vi "APC_init.vi"() -> (0 "error out":errorcluster)   [LabVIEW 2018]
uses:
  <vilib>/Utility/error.llb/Error Cluster From Error Code.vi
  <vilib>/ErrorRing/Error Ring.xnode
panel:
  # "The semaphore handshake with the APC control program is setup\nin a very simple way. A file \"C:\\Users\\Public\\SystemWillShutdown\"\nis created when there is a problem with the power network. This file\nis not deleted by APC control program and must be deleted from\nthis program."
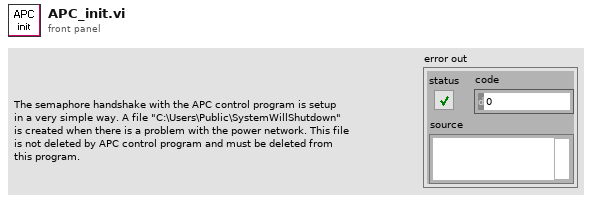
[diagram p1: front panel]
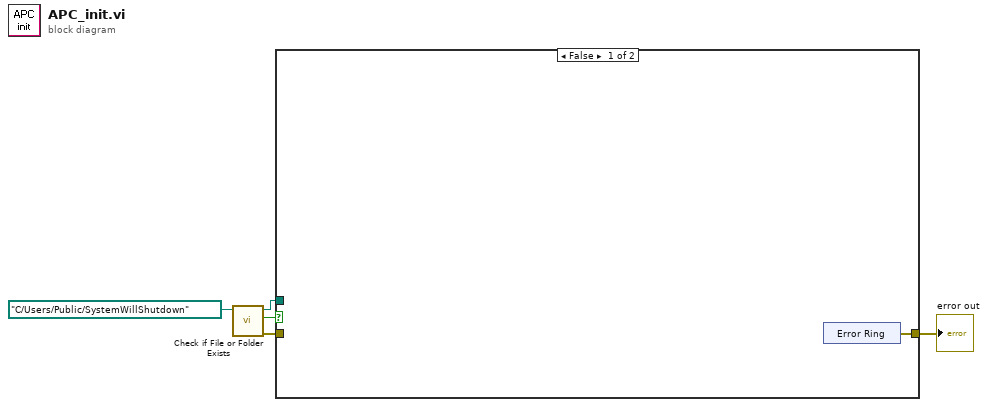
[diagram p0: block diagram]
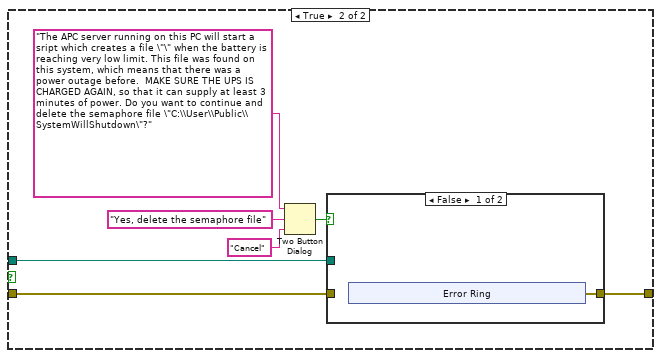
[diagram p2: hidden frame]
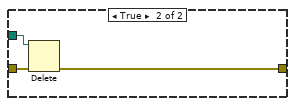
[diagram p3: hidden frame]
diagram:
  n1 = call <vilib>:"Check if File or Folder Exists.vi"("path"=path "C:/Users/Public/SystemWillShutdown" ("path (use dialog)")) -> ("error out"=w3:errorcluster, "file or folder exists?"=w4:bool, "dup path"=w2:path)  [unwired: 8 in]
  n2 = case shown="False" w4 {
    tunnel: w3 -> [_ w9]
    tunnel: w2 -> [_ w10]
    tunnel: [w6 w8] -> w1
    frame False {
      n3 = xnode "Error Ring"() -> ("error out"=w6:errorcluster)
    }
    frame True {
      n4 = Two Button Dialog(message="The APC server running on this PC will start a sript which creates a file \"\" when the battery is reaching very low limit. This file was found on this system, which means that there was a power outage before.  MAKE SURE THE UPS IS CHARGED AGAIN, so that it can supply at least 3 minutes of power. Do you want to continue and delete the semaphore file \"C:\\User\\Public\\SystemWillShutdown\"?", 1:"Cancel" ("F button name (\"Cancel\")"), 2:"Yes, delete the semaphore file" ("T button name (\"OK\")")) -> (T button?=w11:bool)
      n5 = case shown="False" w11 {
        tunnel: w10 -> [_ w23]
        tunnel: w9 -> [_ w22]
        tunnel: [w15 w21] -> w8
        frame False {
          n6 = xnode "Error Ring"() -> ("error out"=w15:errorcluster)
        }
        frame True {
          n7 = Delete(path (use dialog)=w23, error in=w22) -> (error out=w21:errorcluster)  [unwired: 3 in, 2 out]
        }
      }
    }
  }
  "error out" <- w1
